vi "Autosize Cluster.vi"(0 "vi refnum":refnum<vi>, 5 "name":string, 11 "error in":errorcluster) -> (15 "error out":errorcluster)   [LabVIEW 2021, in "Converter Reusables.lvlib"]
uses:
  Converter Reusables.lvlib
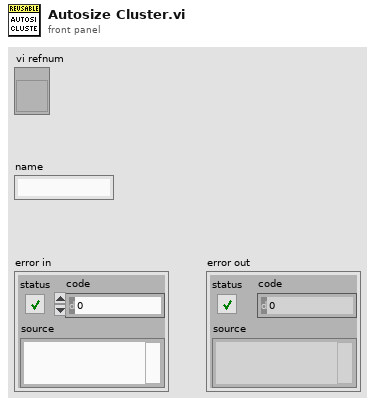
[diagram p1: front panel]
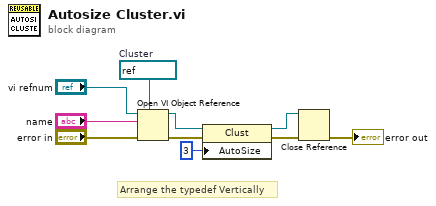
[diagram p0: block diagram]
diagram:
  w3 = refnum<vi> refnum  # Cluster
  # "Arrange the typedef Vertically"
  n1 = Open VI Object Reference(7:w3, 8:"error in", 10:"name", 11:"vi refnum") -> (0:w6:errorcluster, 3:w4:refnum<vi>)
  n2 = property class="Clust"(reference=w4, error in=w6, "AutoSize"=u32 3 ("Auto Sizing")) -> (reference out=w8:refnum<vi>, error out=w7:errorcluster)
  n3 = Close Reference(reference=w8, error in (no error)=w7) -> (error out=→"error out":errorcluster)
